vi "Feeder to Rear Rocket.vi"() -> (4 "path":cluster{"X":dbl, "Y":dbl}[](array[cluster])=[{"X"=16.0, "Y"=25.0}, {"X"=16.99951689536306, "Y"=24.968788753742743}, {"X"=17.99903846961721, "Y"=24.937597482570755}, {"X"=18.998558038807417, "Y"=24.906409086090207}, {"X"=19.998074911955456, "Y"=24.875205425960026}, {"X"=20.997590340857517, "Y"=24.843984062082466}, {"X"=21.997103805097897, "Y"=24.812757164016332}, {"X"=22.99661345405886, "Y"=24.781538634030852}, {"X"=23.996118785883404, "Y"=24.750333323826474}, {"X"=24.99562215541455, "Y"=24.719135892583882}, {"X"=25.99512772674647, "Y"=24.687937107194195}, {"X"=26.994638941665716, "Y"=24.65673088540389}, {"X"=27.994156474544127, "Y"=24.62551720553578}, {"X"=28.993677929522413, "Y"=24.59430038023744}, {"X"=29.993199219688645, "Y"=24.563085261463787}, {"X"=30.992716634695366, "Y"=24.531874307923005}, {"X"=31.992228452288842, "Y"=24.500666937879743}, {"X"=32.991735418646485, "Y"=24.469460802926925}, {"X"=33.991240094537524, "Y"=24.43825366334227}, {"X"=34.990745565800935, "Y"=24.407044639905973}, {"X"=35.99025417378581, "Y"=24.375834335933117}, {"X"=36.98976676509973, "Y"=24.34462407773627}, {"X"=37.98928264204617, "Y"=24.31341491723155}, {"X"=38.988800086167004, "Y"=24.282206994989885}, {"X"=39.98831714368968, "Y"=24.25099953145136}, {"X"=40.98783233828508, "Y"=24.219791337416332}, {"X"=41.98734507906788, "Y"=24.188581500139342}, {"X"=42.98685569033369, "Y"=24.157369879169}, {"X"=43.98636513420301, "Y"=24.126157195372738}, {"X"=44.98587458258912, "Y"=24.094944713648793}, {"X"=45.98538500790048, "Y"=24.063733697956675}, {"X"=46.98489691723439, "Y"=24.032524890472324}, {"X"=47.98441028174495, "Y"=24.001318225469884}, {"X"=48.98392464155813, "Y"=23.970112870264263}, {"X"=49.983439318428736, "Y"=23.938907549378566}, {"X"=50.98295365177674, "Y"=23.907701008123507}, {"X"=51.982467185608364, "Y"=23.876492438385128}, {"X"=52.981979763505116, "Y"=23.845281723418996}, {"X"=53.98149152355554, "Y"=23.81406943694362}, {"X"=54.98100281402169, "Y"=23.782856620928452}, {"X"=55.98051406732171, "Y"=23.75164443496216}, {"X"=56.98002567310077, "Y"=23.720433799168873}, {"X"=57.97953788318582, "Y"=23.689225139536372}, {"X"=58.97905076671606, "Y"=23.658018300147678}, {"X"=59.9785642178027, "Y"=23.626812629670034}, {"X"=60.97807800487347, "Y"=23.595607198509818}, {"X"=61.977591842921626, "Y"=23.564401071981703}, {"X"=62.97710546790033, "Y"=23.533193559148266}, {"X"=63.97661869567063, "Y"=23.50198437403244}, {"X"=64.97613145443962, "Y"=23.47077367729137}, {"X"=65.97564378740284, "Y"=23.439562001464235}, {"X"=66.9751558293855, "Y"=23.408350091884007}, {"X"=67.97466776629764, "Y"=23.377138711935515}, {"X"=68.97417978849909, "Y"=23.345928463510955}, {"X"=69.97369204874911, "Y"=23.314719663149894}, {"X"=70.97320463286319, "Y"=23.283512296032193}, {"X"=71.97271754740851, "Y"=23.25230604932184}, {"X"=72.97223072470489, "Y"=23.22110040845692}, {"X"=73.9717440419078, "Y"=23.189894788393868}, {"X"=74.97125734861636, "Y"=23.158688668038064}, {"X"=75.97077049652378, "Y"=23.127481699657164}, {"X"=76.97028336506742, "Y"=23.09627377402511}, {"X"=77.96979587853316, "Y"=23.065065033664546}, {"X"=78.9693080121886, "Y"=23.033855838060802}, {"X"=79.96881978727492, "Y"=23.002646693842493}, {"X"=80.96833125665702, "Y"=22.97143816826497}, {"X"=81.96784248429677, "Y"=22.940230805459386}, {"X"=82.96735352233301, "Y"=22.909025062275525}, {"X"=83.96686438940704, "Y"=22.877821275221095}, {"X"=84.96637505310215, "Y"=22.84661966339055}, {"X"=85.96588541816826, "Y"=22.815420365786007}, {"X"=86.96539532083023, "Y"=22.78422350623785}, {"X"=87.96490452816566, "Y"=22.753029276001868}, {"X"=88.96441274047092, "Y"=22.72183802334422}, {"X"=89.96391959383583, "Y"=22.690650340892237}, {"X"=90.96342465985595, "Y"=22.659467144745683}, {"X"=91.96292743948733, "Y"=22.62828974362655}, {"X"=92.96242734840833, "Y"=22.59711990095555}, {"X"=93.96192369175182, "Y"=22.56595989702079}, {"X"=94.9614156265645, "Y"=22.534812601874467}, {"X"=95.96090211069615, "Y"=22.503681572024103}, {"X"=96.96038183689642, "Y"=22.47257118540442}, {"X"=97.95985315060732, "Y"=22.441486829780693}, {"X"=98.95931394924257, "Y"=22.41043516008073}, {"X"=99.95876155960536, "Y"=22.379424440722637}, {"X"=100.9581925885223, "Y"=22.348464990376623}, {"X"=101.95760273976366, "Y"=22.31756974933183}, {"X"=102.9569865878803, "Y"=22.286754994226765}, {"X"=103.95633729668263, "Y"=22.2560412317796}, {"X"=104.95564626665866, "Y"=22.225454312694083}, {"X"=105.95490269153812, "Y"=22.195026819485456}, {"X"=106.9540929992902, "Y"=22.164799797979864}, {"X"=107.95320014681595, "Y"=22.134824922225505}, {"X"=108.9522027301184, "Y"=22.10516720725338}, {"X"=109.95107386237012, "Y"=22.07590841456526}, {"X"=110.94977976048479, "Y"=22.04715133281434}, {"X"=111.94827796586166, "Y"=22.019025162750463}, {"X"=112.9465151060733, "Y"=21.991692293575504}, {"X"=113.94442408036386, "Y"=21.965356830525895}, {"X"=114.94192052165133, "Y"=21.940275324731285}, {"X"=115.93889834967443, "Y"=21.91677027116779}, {"X"=116.93522418201573, "Y"=21.895247085047636}, {"X"=117.93073030945604, "Y"=21.87621544903458}, {"X"=118.92520586634097, "Y"=21.86031615294628}, {"X"=119.91838573139285, "Y"=21.84835483624327}, {"X"=120.90993657479753, "Y"=21.841344406827435}, {"X"=121.89943931645242, "Y"=21.84055836645048}, {"X"=122.88636707447505, "Y"=21.847597848378804}, {"X"=123.87005743085999, "Y"=21.864475890482762}, {"X"=124.84967759557475, "Y"=21.89372339653579}, {"X"=125.82418052119392, "Y"=21.938522303429988}, {"X"=126.79224990710365, "Y"=22.00287312250271}, {"X"=127.75223077006247, "Y"=22.091805342648644}, {"X"=128.7020424895756, "Y"=22.211642307664896}, {"X"=129.63906922376754, "Y"=22.370333864361285}, {"X"=130.57229216062453, "Y"=22.577491693211083}, {"X"=131.5024895771261, "Y"=22.823199452101672}, {"X"=132.43028052717784, "Y"=23.099569702419394}, {"X"=133.3561573935105, "Y"=23.40032876785482}, {"X"=134.28051181171665, "Y"=23.72048658441299}, {"X"=135.2036552973393, "Y"=24.056074075763213}, {"X"=136.12583563317597, "Y"=24.403934234348682}, {"X"=137.04724989667355, "Y"=24.761555964986158}, {"X"=137.9680548328992, "Y"=25.12694194812247}, {"X"=138.8883751133868, "Y"=25.498503534041777}, {"X"=139.8083099013658, "Y"=25.87497712440227}, {"X"=140.72793806695032, "Y"=26.255357657959866}, {"X"=141.64732233495033, "Y"=26.638845714580032}, {"X"=142.56651258889227, "Y"=27.024805448298682}, {"X"=143.48554850242365, "Y"=27.41273112252535}, {"X"=144.40446163116638, "Y"=27.80222048273558}, {"X"=145.32327707327414, "Y"=28.1929535728421}, {"X"=146.24201478848718, "Y"=28.584675888503224}, {"X"=147.16069064809784, "Y"=28.97718498160897}, {"X"=148.07931727165973, "Y"=29.3703198060795}, {"X"=148.9979046927702, "Y"=29.763952240069564}, {"X"=149.91646088713773, "Y"=30.15798033876853}, {"X"=150.8349921904311, "Y"=30.552322966224416}, {"X"=151.753503629068, "Y"=30.946915526465624}, {"X"=152.67199918275782, "Y"=31.34170656895082}, {"X"=153.59048199316993, "Y"=31.73665508699745}, {"X"=154.50895452928293, "Y"=32.13172836431064}, {"X"=155.42741871732085, "Y"=32.526900255385776}, {"X"=156.34587604167095, "Y"=32.92214981021865}, {"X"=157.2643276222679, "Y"=33.31746017241575}, {"X"=158.18277427306026, "Y"=33.71281769340465}, {"X"=159.10121654507896, "Y"=34.108211215633595}, {"X"=160.01965475642402, "Y"=34.503631485931756}, {"X"=160.93808901041038, "Y"=34.899070667357286}, {"X"=161.85651920235486, "Y"=35.294521923915255}, {"X"=162.77494501503003, "Y"=35.689979057148214}, {"X"=163.69336590248056, "Y"=36.08543617656852}, {"X"=164.61178106150672, "Y"=36.48088738733308}, {"X"=165.53018938951644, "Y"=36.87632647885203}, {"X"=166.44858942664024, "Y"=37.271746597581135}, {"X"=167.36697927902856, "Y"=37.66713988628559}, {"X"=168.28535651915854, "Y"=38.06249707049643}, {"X"=169.20371805778308, "Y"=38.457806970429395}, {"X"=170.1220599807454, "Y"=38.85305591293023}, {"X"=171.0403773421614, "Y"=39.24822701274594}, {"X"=171.95866390324417, "Y"=39.643299285340724}, {"X"=172.87691180320135, "Y"=40.03824654435188}, {"X"=173.79511114499653, "Y"=40.433036025267405}, {"X"=174.7132494742038, "Y"=40.827626662492825}, {"X"=175.63131112348105, "Y"=41.22196692887452}, {"X"=176.5492763880851, "Y"=41.61599212393451}, {"X"=177.46712048896606, "Y"=42.009620968241805}, {"X"=178.3848122688306, "Y"=42.402751324913304}, {"X"=179.3023125525462, "Y"=42.795254823273666}, {"X"=180.2195720856067, "Y"=43.186970101829274}, {"X"=181.13652894216906, "Y"=43.5776943149383}, {"X"=182.05310526622247, "Y"=43.967172456111555}, {"X"=182.96920317433265, "Y"=44.35508393596133}, {"X"=183.88469960424348, "Y"=44.74102570836935}, {"X"=184.79943983828767, "Y"=45.124491056891564}, {"X"=185.71322935966825, "Y"=45.50484292460913}, {"X"=186.62582361888775, "Y"=45.88128038602824}, {"X"=187.53691514548376, "Y"=46.252796487115276}, {"X"=188.44611741916145, "Y"=46.618125265987324}, {"X"=189.35294439210176, "Y"=46.97567508179891}, {"X"=190.2567851661074, "Y"=47.32344492015316}, {"X"=191.15687146202902, "Y"=47.65891897781893}, {"X"=192.05223757365474, "Y"=47.97893433988644}, {"X"=192.9416693091186, "Y"=48.27951447730135}, {"X"=193.84810694566656, "Y"=48.566197789714785}, {"X"=194.76807074027357, "Y"=48.84182649950043}, {"X"=195.69879286574974, "Y"=49.108661020402586}, {"X"=196.63807167421513, "Y"=49.3684989063184}, {"X"=197.5841558650546, "Y"=49.62276946056508}, {"X"=198.53565234786913, "Y"=49.87260897585319}, {"X"=199.4914528953029, "Y"=50.118920539712796}, {"X"=200.45067578720275, "Y"=50.36242155595603}, {"X"=201.41261941608872, "Y"=50.60368149943173}, {"X"=202.376725383795, "Y"=50.843151893677664}, {"X"=203.34254911297882, "Y"=51.08119007968719}, {"X"=204.309736432255, "Y"=51.31807802123594}, {"X"=205.27800492693655, "Y"=51.554037140368315}, {"X"=206.24712908203662, "Y"=51.789239969717656}, {"X"=207.21692842374347, "Y"=52.0238192356962}, {"X"=208.18725802267082, "Y"=52.257874846979796}, {"X"=209.15800085920486, "Y"=52.491479153096535}, {"X"=210.1290616579911, "Y"=52.72468075032929}, {"X"=211.1003618733739, "Y"=52.95750703774221}, {"X"=212.07183556035505, "Y"=53.189965659502775}, {"X"=213.04342590800783, "Y"=53.42204490890078}, {"X"=214.01508224922438, "Y"=53.65371311365356}, {"X"=214.98675739046075, "Y"=53.884916969025404}, {"X"=215.9584051245906, "Y"=54.11557873127389}, {"X"=216.9299777985558, "Y"=54.345592124799985}, {"X"=217.90142380751107, "Y"=54.57481674847086}, {"X"=218.8726848813493, "Y"=54.80307068675402}, {"X"=219.84369301877462, "Y"=55.03012093613027}, {"X"=220.81436690721577, "Y"=55.25567114220117}, {"X"=221.78460764132305, "Y"=55.479346001822016}, {"X"=222.75429351623177, "Y"=55.70067150960169}, {"X"=223.72327362238212, "Y"=55.91905000964665}, {"X"=224.69135990363057, "Y"=56.13372873972195}, {"X"=225.65831726405307, "Y"=56.343760212854455}, {"X"=226.62385118231757, "Y"=56.54795234875742}, {"X"=227.58759225031176, "Y"=56.74480573583566}, {"X"=228.5490766300072, "Y"=56.93243471110367}, {"X"=229.5077218318638, "Y"=57.1084681138223}, {"X"=230.46279577822767, "Y"=57.26992450178991}, {"X"=231.41337856026644, "Y"=57.413055198200084}, {"X"=232.358313853157, "Y"=57.53314703744902}, {"X"=233.31451144088714, "Y"=57.62866767492872}, {"X"=234.27966594617058, "Y"=57.704644502705136}, {"X"=235.25194341946874, "Y"=57.76507630138647}, {"X"=236.2298847691108, "Y"=57.81314369914958}, {"X"=237.21232899839632, "Y"=57.85137655781264}, {"X"=238.19835212766384, "Y"=57.88178712695768}, {"X"=239.18721854474865, "Y"=57.90597596273661}, {"X"=240.1783422679181, "Y"=57.92521616635259}, {"X"=241.1712561131954, "Y"=57.94052038104107}, {"X"=242.1655871229408, "Y"=57.952694087676484}, {"X"=243.1610369372555, "Y"=57.96237800443682}, {"X"=244.15736607879654, "Y"=57.97008181265322}, {"X"=245.15438134183066, "Y"=57.97621097956193}, {"X"=246.15192562824373, "Y"=57.98108809418377}, {"X"=247.14986968712955, "Y"=57.98496984481794}, {"X"=248.14810531387423, "Y"=57.988060531819535}, {"X"=249.14653965058872, "Y"=57.99052282294488}, {"X"=250.1450902942226, "Y"=57.992486314564786}, {"X"=251.14368095953606, "Y"=57.994054350192656}, {"X"=252.14223746768, "Y"=57.99530945790593}, {"X"=253.1406838451122, "Y"=57.99631769435872}, {"X"=254.13893832483495, "Y"=57.99713212323518}, {"X"=255.13690904023565, "Y"=57.99779560937397}, {"X"=256.1344891875679, "Y"=57.99834307456421}, {"X"=257.13155140441137, "Y"=57.99880333418909}, {"X"=258.1279410680653, "Y"=57.99920061264918}, {"X"=259.12346815950946, "Y"=57.99955581822957}, {"X"=260.11789726318136, "Y"=57.99988764442723}, {"X"=261.11093517590325, "Y"=58.000213554897314}, {"X"=262.1022154738002, "Y"=58.00055070306165}, {"X"=263.0912792248088, "Y"=58.000916834556726}, {"X"=264.077550839574, "Y"=58.00133122040558}, {"X"=265.0603077570435, "Y"=58.00181567064296}, {"X"=266.0386424822742, "Y"=58.002395682130334}, {"X"=267.0114146601069, "Y"=58.003101780928645}, {"X"=267.97719137021073, "Y"=58.00397112951788}, {"X"=268.9341712553163, "Y"=58.005049483062656}, {"X"=269.88009017556715, "Y"=58.00639359751039}, {"X"=270.8121017744606, "Y"=58.00807421637194}, {"X"=271.757555488075, "Y"=58.010179793656036}, {"X"=272.7135804763675, "Y"=58.01282114914891}, {"X"=273.677862301875, "Y"=58.016137301138066}, {"X"=274.64852104190084, "Y"=58.02030278346613}, {"X"=275.62401239418574, "Y"=58.0255368318262}, {"X"=276.60304644287044, "Y"=58.032114922617545}, {"X"=277.5845197385209, "Y"=58.040383271614076}, {"X"=278.567457187103, "Y"=58.05077705560397}, {"X"=279.5509607410946, "Y"=58.06384331617619}, {"X"=280.5341621617633, "Y"=58.08026975124557}, {"X"=281.5161773252859, "Y"=58.10092090972512}, {"X"=282.4960596705296, "Y"=58.12688369419554}, {"X"=283.4727503734768, "Y"=58.15952456706544}, {"X"=284.44502260715683, "Y"=58.200561467049724}, {"X"=285.41141704521027, "Y"=58.25215423758672}, {"X"=286.37016490907234, "Y"=58.31701827131769}, {"X"=287.319095150549, "Y"=58.39856749749829}, {"X"=288.25551977225297, "Y"=58.50109393605625}, {"X"=289.1760927614421, "Y"=58.629993754117606}, {"X"=290.0766337607418, "Y"=58.79205114289301}, {"X"=290.9812080847602, "Y"=58.99579541833576}, {"X"=291.8885577313262, "Y"=59.23240310411671}, {"X"=292.7975707889964, "Y"=59.49478036584945}, {"X"=293.70722284415484, "Y"=59.77718963971381}, {"X"=294.61652309567626, "Y"=60.07494768947142}, {"X"=295.5244622764677, "Y"=60.384179127834244}, {"X"=296.4299594533817, "Y"=60.701612419996174}, {"X"=297.3318052228391, "Y"=61.02440769178737}, {"X"=298.2285978937018, "Y"=61.35000729396134}, {"X"=299.118669913879, "Y"=61.676001159782146}, {"X"=300.0, "Y"=62.0}], 6 "Reverse Path?":bool=TRUE)   [LabVIEW 2018]
uses:
  AutonBuilder/Typedef/Data Point.ctl
panel:
  in  "Data Points":T1[](array[typedef])=[{"X"=16.0, "Y"=25.0, "Theta"=0.0, "Speed %"=0.0, "Disabled?"=FALSE}, {"X"=129.71134020618558, "Y"=21.44947735191638, "Theta"=0.0, "Speed %"=0.0, "Disabled?"=FALSE}, {"X"=192.61855670103094, "Y"=48.54355400696864, "Theta"=0.0, "Speed %"=0.0, "Disabled?"=FALSE}, {"X"=232.14432989690724, "Y"=58.0, "Theta"=0.0, "Speed %"=0.0, "Disabled?"=FALSE}, {"X"=270.55670103092785, "Y"=58.0, "Theta"=0.0, "Speed %"=0.0, "Disabled?"=FALSE}, {"X"=290.0, "Y"=58.0, "Theta"=0.0, "Speed %"=0.0, "Disabled?"=FALSE}, {"X"=300.0, "Y"=62.0, "Theta"=0.0, "Speed %"=0.0, "Disabled?"=FALSE}]
  out "Graph":cluster{dbl[], dbl[]}[](graph)=[{[-3.5, 30.0, 30.0, -3.5, -3.5], [39.25, 39.25, 10.75, 10.75, 39.25]}, {[16.0, 129.71134020618558, 192.61855670103094, 232.14432989690724, 270.55670103092785, 290.0, 300.0], [25.0, 21.44947735191638, 48.54355400696864, 58.0, 58.0, 58.0, 62.0]}, {array[295 elements], array[295 elements]}, {array[295 elements], array[295 elements]}, {array[295 elements], array[295 elements]}, {[], []}, {[], []}, {[], []}, {[], []}, {[], []}, {[], []}, {[], []}, {[], []}, {[], []}, {[], []}, {[], []}, {[], []}, {[], []}, {[], []}, {[], []}]
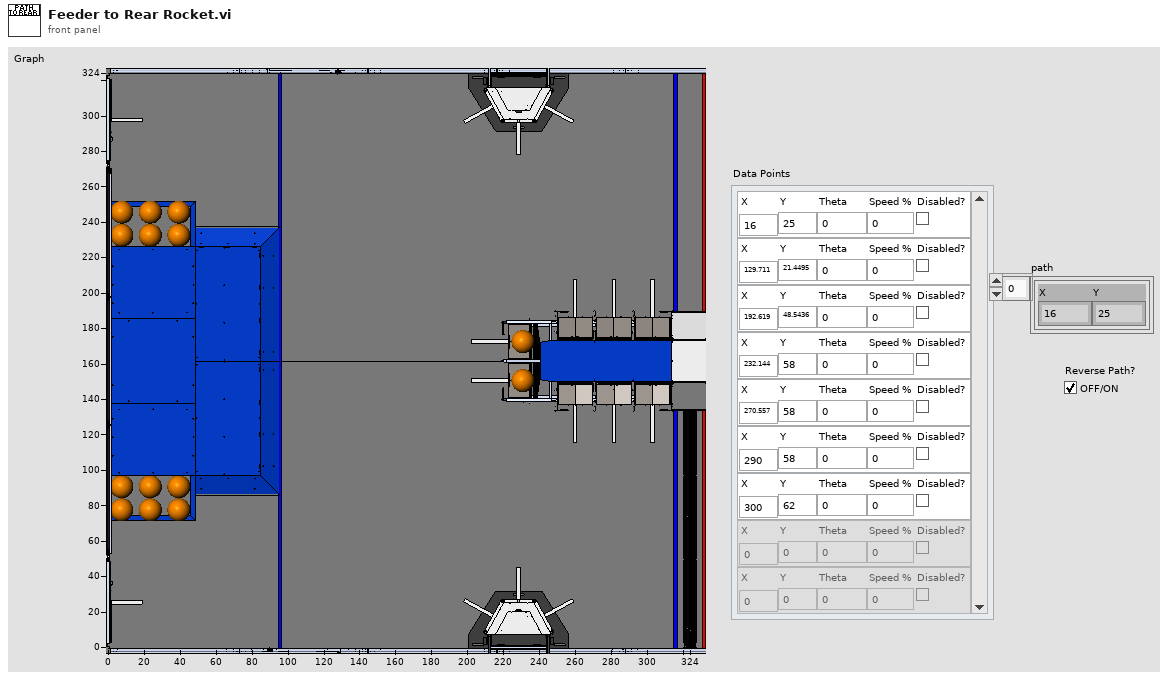
[diagram p1: front panel]
types:
  T1 = typedef "Data Point.ctl" = cluster{"X":dbl, "Y":dbl, "Theta":dbl, "Speed %":dbl, "Disabled?":bool}
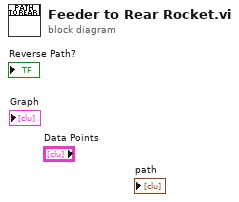
[diagram p0: block diagram]
diagram:
